vi "Write Test Finder.vi"(8 "error in (no error)":errorcluster, 10 "Test Finder.lvclass":refnum<class "Test Finder.lvclass">, 11 "Test Finder In":refnum<class "Test Finder Test.lvclass">) -> (0 "error out":errorcluster, 3 "Test Finder Out":refnum<class "Test Finder Test.lvclass">)   [LabVIEW 2020, in "LUnit Tests.lvlib" / "Test Finder Test.lvclass"]
uses:
  Test Finder Test.lvclass
  source/Framework/Helper Classes/Test Finder/Test Finder.lvclass
  Test Finder Test.lvclass/Test Finder Test.ctl
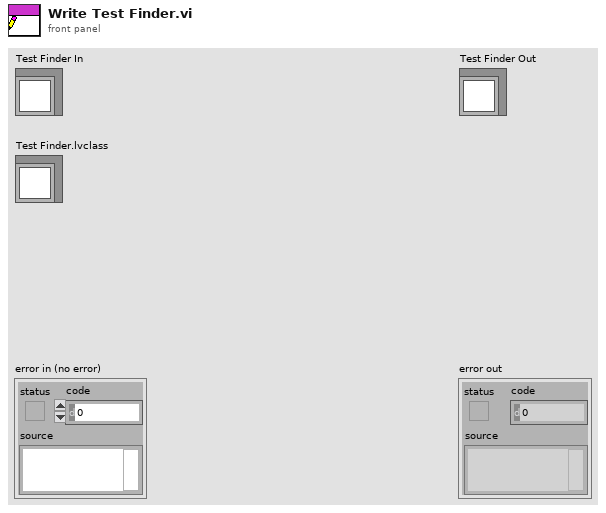
[diagram p1: front panel]
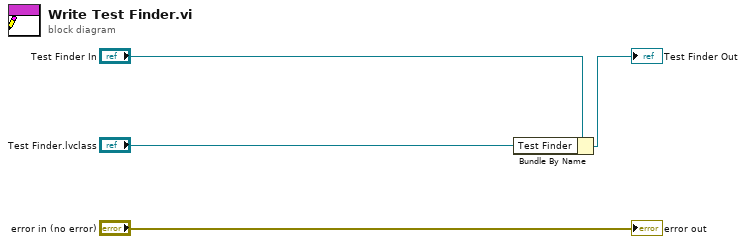
[diagram p0: block diagram]
diagram:
  n1 = Bundle By Name(cluster="Test Finder In", "Test Finder"="Test Finder.lvclass") -> (→"Test Finder Out":refnum<class "Test Finder Test.lvclass">)
  "error out" <- "error in (no error)"
